vi "Write pretty.vi"(10 "pretty":bool, 11 "StringFormatter in":refnum<class "StringFormatter.lvclass">) -> (3 "StringFormatter out":refnum<class "StringFormatter.lvclass">)   [LabVIEW 2013, in "OpenStringFormatter.lvlib" / "StringFormatter.lvclass"]
uses:
  StringFormatter.lvclass
  StringFormatter.lvclass/StringFormatter.ctl
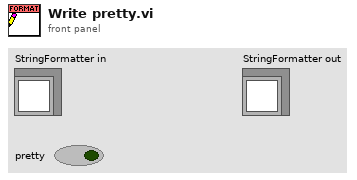
[diagram p1: front panel]
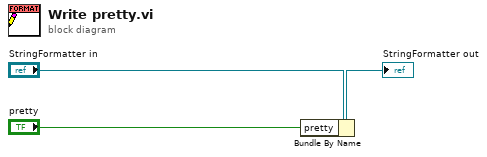
[diagram p0: block diagram]
diagram:
  n1 = Bundle By Name(cluster="StringFormatter in", "pretty"="pretty") -> (→"StringFormatter out":refnum<class "StringFormatter.lvclass">)
